vi "DP-Create Tones.vi"(1 "f1":dbl, 2 "f2":dbl, 5 "Sampling rate (Hz)":dbl, 7 "Npts":i32, 9 "AO channels":u16[](array[numeric]), 11 "error in (no error)":errorcluster) -> (8 "stimuli":dbl[][](array[numeric]), 15 "error out":errorcluster)   [LabVIEW 2020]
uses:
  epl-vi-lib/PXI DAQ VIs/DAQ Engine VIs/PXI Globals.vi
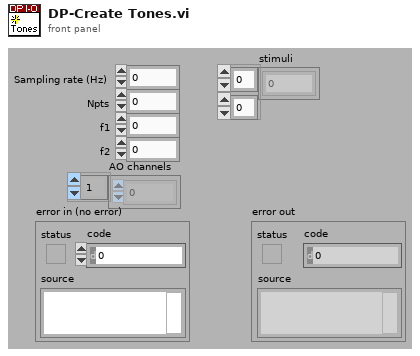
[diagram p1: front panel]
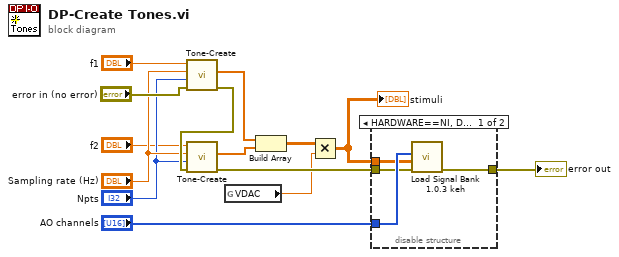
[diagram p0: block diagram]
diagram:
  n1 = call "Tone-Create.vi"("error in (no error)"="error in (no error)", "Npts"="Npts", "Sampling Rate (Hz)"="Sampling rate (Hz)", "Frequency (kHz)"="f1") -> ("error out"=w14:errorcluster, "Waveform"=w11:dbl[])  [unwired: 6 in]
  n2 = call "Tone-Create.vi"("error in (no error)"=w14, "Npts"="Npts", "Sampling Rate (Hz)"="Sampling rate (Hz)", "Frequency (kHz)"="f2") -> ("error out"=w8:errorcluster, "Waveform"=w10:dbl[])  [unwired: 6 in]
  n3 = global read "PXI Globals.vi" "VDAC"() -> (w4:dbl)
  n4 = Build Array(w11, w10) -> (w7:dbl[][])
  n5 = Multiply(x=w7, y=w4) -> (x*y=w3:dbl[][])
  "stimuli" <- w3
  n6 = disable-structure shown="HARDWARE==NI, Default" {
    disable-tunnel: "AO channels" -> [w18 _]
    disable-tunnel: [w17 w19] -> w12
    disable-tunnel: w8 -> [w16 w19]
    disable-tunnel: w3 -> [w15 _]
    frame condition #0 (active) {
      n7 = call "Load Signal Bank 1.0.3 keh.vi"("error in (no error)"=w16, "Input array"=w15, "Active AO Array"=w18) -> ("error out"=w17:errorcluster)  [unwired: 6 in, 2 out]
    }
    frame condition #1 {
    }
  }
  "error out" <- w12
